vi "Set Cell Text.vi"(7 "Sheet Name":string="table2", 8 "error in (no error)":errorcluster, 9 "position":cluster{"Row":i32, "Column":i32}={"Row"=1, "Column"=1}, 10 "text":string, 11 "report in":refnum<class "ooCalc.lvclass">) -> (0 "error out":errorcluster, 3 "report out":refnum<class "ooCalc.lvclass">)   [LabVIEW 2009, in "ooCalc.lvclass"]
doc: "Appends text to the selected report."
uses:
  ooCalc.lvclass
  ooCalc.lvclass/ooCalc.ctl
  C:/Projets/LAVAG/OpenOfficeRGT/AODL/DLLs/AODL.dll
panel:
  in  "Value":variant
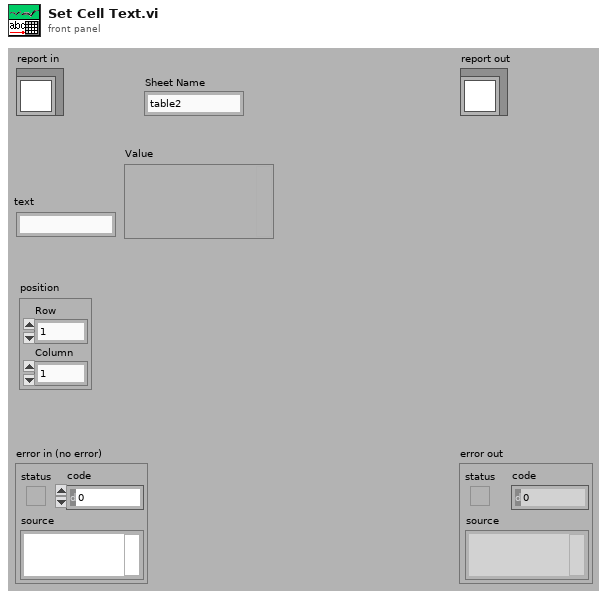
[diagram p1: front panel]
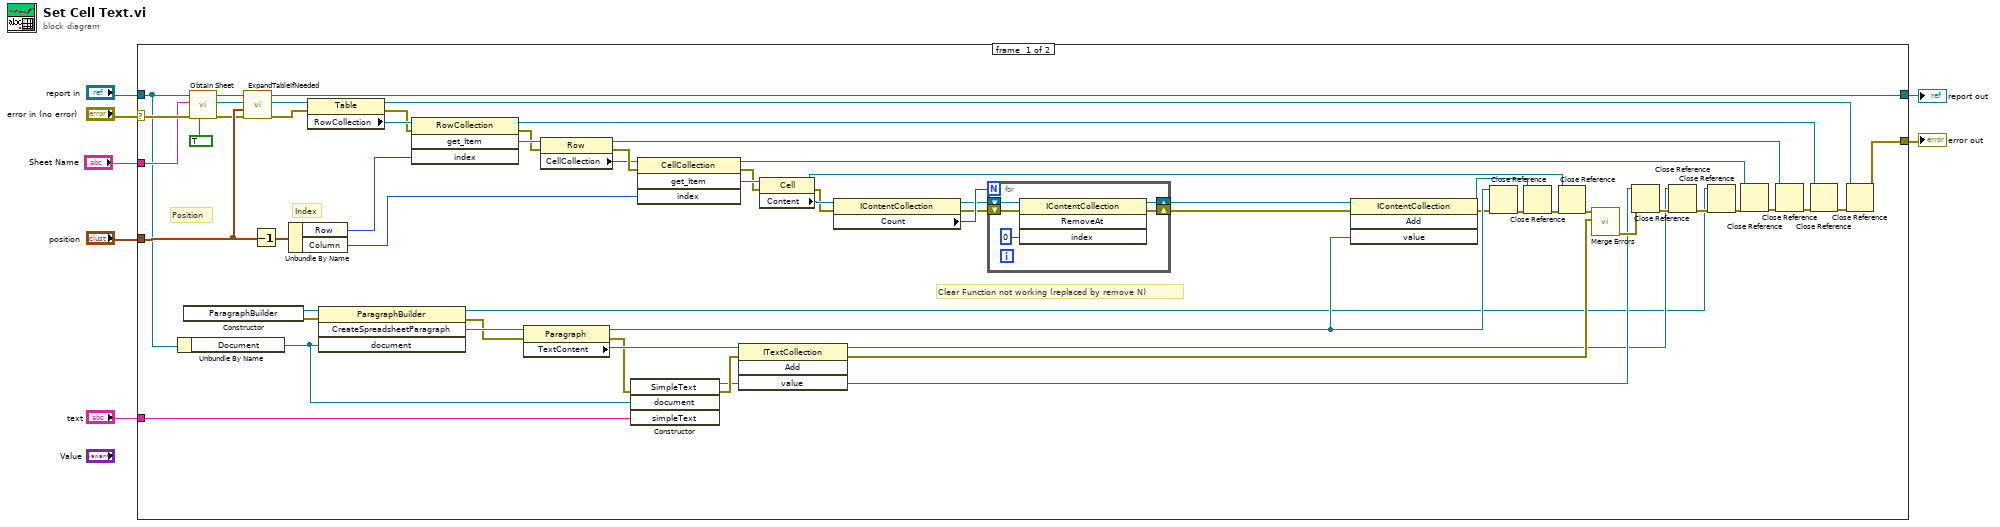
[diagram p0: block diagram]
diagram:
  n1 = case shown="No Error" "error in (no error)" {
    selector: "error in (no error)" -> [w67 w74]
    tunnel: [w18 w74] -> w5
    tunnel: [w56 w73] -> w6
    tunnel: "report in" -> [w43 w73]
    tunnel: "text" -> [w12 _]
    tunnel: "Sheet Name" -> [w62 _]
    tunnel: "position" -> [w52 _]
    frame #0 {
      # "Clear Function not working (replaced by remove N)"
      # "Position"
      # "Index"
      n2 = Unbundle By Name(w43) -> ("Document"=w61:refnum<k24>)
      n3 = constructor class="ParagraphBuilder"() -> (reference out=w65:refnum<k24>, error out=w66:errorcluster)  [unwired: 3 in, 1 out]
      n4 = call-dynamic "Obtain Sheet.vi"("Create if non-existant? (T)"=TRUE, "error in (no error)"=w67, "Sheet Name"=w62, "ooCalc in"=w43) -> ("error out"=w44:errorcluster, "Sheet"=w59:refnum<k24>, "ooCalc out"=w56:refnum<class "ooCalc.lvclass">)  [unwired: 5 in]
      n5 = call "ExpandTableIfNeeded.vi"("error in"=w44, "Table Size"=w52, "Table in"=w59) -> ("error out"=w48:errorcluster, "Table out"=w55:refnum<k24>)  [unwired: 7 in]
      n6 = Decrement(x=w52) -> (x-1=w45:cluster{"Row":i32, "Column":i32})
      n7 = Unbundle By Name(w45) -> ("Row"=w50:i32, "Column"=w51:i32)
      n8 = property on="Property Node" class="Table"(reference=w55, error in=w48) -> (reference out=w19:refnum<k24>, error out=w53:errorcluster, "RowCollection"=w54:refnum<k24>)
      n9 = invoke class="ParagraphBuilder" method="CreateSpreadsheetParagraph"(reference=w65, error in=w66, "document"=w61) -> (reference out=w27:refnum<k24>, error out=w36:errorcluster, "CreateSpreadsheetParagraph"=w64:refnum<k24>)  [unwired: 1 in, 1 out]
      n10 = invoke class="RowCollection" method="get_Item"(reference=w54, error in=w53, "index"=w50) -> (reference out=w21:refnum<k24>, error out=w46:errorcluster, "get_Item"=w49:refnum<k24>)  [unwired: 1 in, 1 out]
      n11 = property on="Property Node" class="Paragraph"(reference=w64, error in=w36) -> (reference out=w41:refnum<k24>, error out=w35:errorcluster, "TextContent"=w63:refnum<k24>)
      n12 = property on="Property Node" class="Row"(reference=w49, error in=w46) -> (reference out=w22:refnum<k24>, error out=w47:errorcluster, "CellCollection"=w42:refnum<k24>)
      n13 = constructor class="SimpleText"(error in=w35, "document"=w61, "simpleText"=w12) -> (reference out=w30:refnum<k24>, error out=w34:errorcluster)  [unwired: 2 in, 3 out]
      n14 = invoke class="CellCollection" method="get_Item"(reference=w42, error in=w47, "index"=w51) -> (reference out=w23:refnum<k24>, error out=w57:errorcluster, "get_Item"=w58:refnum<k24>)  [unwired: 1 in, 1 out]
      n15 = invoke class="ITextCollection" method="Add"(reference=w63, error in=w34, "value"=w30) -> (reference out=w29:refnum<k24>, error out=w32:errorcluster)  [unwired: 1 in, 2 out]
      n16 = property on="Property Node" class="Cell"(reference=w58, error in=w57) -> (reference out=w9:refnum<k24>, error out=w13:errorcluster, "Content"=w16:refnum<k24>)
      n17 = property on="Property Node" class="IContentCollection"(reference=w16, error in=w13) -> (reference out=w15:refnum<k24>, error out=w14:errorcluster, "Count"=w17:i32)
      n18 = for {
        N: w17 -> [_]
        shift-right: [w72] -> w11
        shift-left: w15 -> [w69]
        shift-right: [w71] -> w10
        shift-left: w14 -> [w70]
        n19 = invoke class="IContentCollection" method="RemoveAt"(reference=w69, error in=w70, "index"=0) -> (reference out=w72:refnum<k24>, error out=w71:errorcluster)  [unwired: 1 in, 2 out]
      }
      n20 = invoke class="IContentCollection" method="Add"(reference=w11, error in=w10, "value"=w41) -> (reference out=w37:refnum<k24>, error out=w8:errorcluster)  [unwired: 1 in, 2 out]
      n21 = Close Reference(reference=w41, error in (no error)=w8) -> (error out=w40:errorcluster)
      n22 = Close Reference(reference=w37, error in (no error)=w40) -> (error out=w38:errorcluster)
      n23 = Close Reference(reference=w9, error in (no error)=w38) -> (error out=w33:errorcluster)
      n24 = call <vilib>:"Merge Errors.vi"("error in 2 (no error)"=w32, "error in 1 (no error)"=w33) -> ("error out"=w31:errorcluster)  [unwired: 5 in]
      n25 = Close Reference(reference=w30, error in (no error)=w31) -> (error out=w39:errorcluster)
      n26 = Close Reference(reference=w29, error in (no error)=w39) -> (error out=w28:errorcluster)
      n27 = Close Reference(reference=w27, error in (no error)=w28) -> (error out=w24:errorcluster)
      n28 = Close Reference(reference=w23, error in (no error)=w24) -> (error out=w26:errorcluster)
      n29 = Close Reference(reference=w22, error in (no error)=w26) -> (error out=w25:errorcluster)
      n30 = Close Reference(reference=w21, error in (no error)=w25) -> (error out=w20:errorcluster)
      n31 = Close Reference(reference=w19, error in (no error)=w20) -> (error out=w18:errorcluster)
    }
    frame #1 {
    }
  }
  "error out" <- w5
  "report out" <- w6
